vi "Get SSR Status - Multiple.vi"(0 "reference in":refnum<class "SSR.lvclass">, 3 "SSR Channel Numbers (Zero Based)":i32[](array[numeric]), 5 "error in (no error)":errorcluster) -> (14 "reference out":refnum<class "SSR.lvclass">, 17 "SSR Channel Status":bool[](array[boolean]), 19 "error out":errorcluster)   [LabVIEW 2017, in "SSR.lvclass"]
uses:
  SSR.lvclass
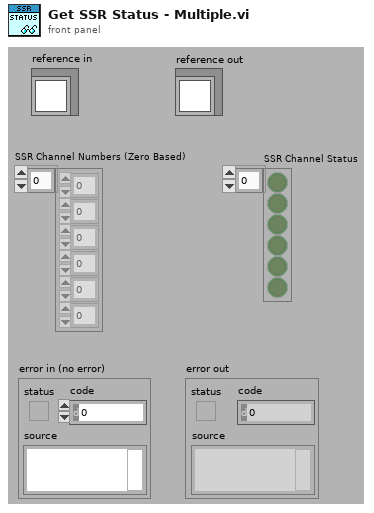
[diagram p1: front panel]
types:
  T1 = typedef "SSR.lvclass/ObjectAttributes.ctl" = cluster{"SSR Task":refnum<k21>, "SSR On/Off Status":bool, "Number of SSR Modules":u32, "Number of Total SSR Channels":u32, "SSR Module Names (NI-Max Name)":string[], "Number of Channels Per SSR Module":i32[], "SSR Status":bool[], "SSR Status to Set":bool[], "SSR VI Reference":refnum<vi>}
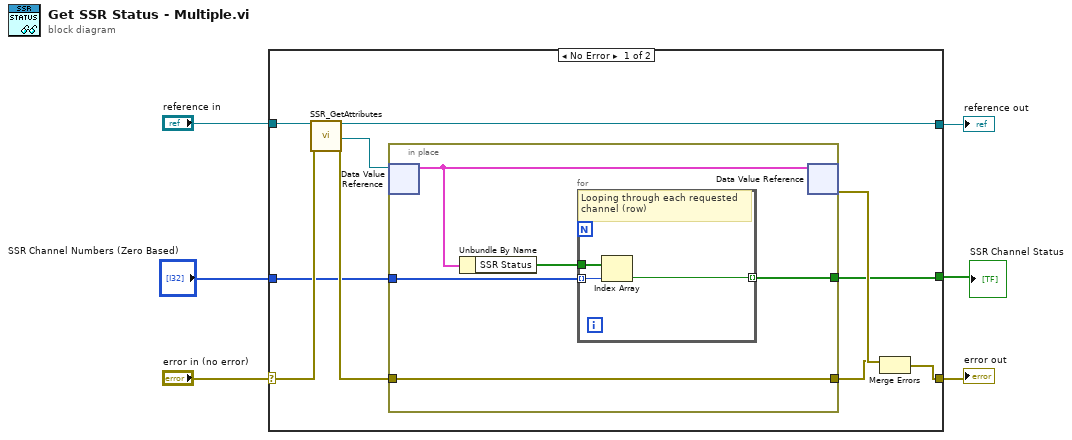
[diagram p0: block diagram]
diagram:
  n1 = case shown="No Error" "error in (no error)" {
    selector: "error in (no error)" -> [w15 w26]
    tunnel: [w12 w26] -> w5
    tunnel: [w13 w25] -> w3
    tunnel: "reference in" -> [w16 w25]
    tunnel: "SSR Channel Numbers (Zero Based)" -> [w8 _]
    tunnel: [w7 _] -> w1
    frame No Error {
      n2 = call "SSR_GetAttributes.vi"("reference in"=w16, "error in (no error)"=w15) -> ("reference out"=w13:refnum<class "SSR.lvclass">, "DataRef"=w11:refnum<data-value>, "error out"=w10:errorcluster)  [unwired: 14 in, 1 out]
      n3 = in-place {
        in-place-border: w10 -> [w21]
        in-place-border: [w21] -> w9
        in-place-border: w8 -> [w18]
        in-place-border: [w17] -> w7
        n4 = in-place-dvr #1(w11) -> (w20:T1)  [unwired: 1 out]
        n5 = Unbundle By Name(w20) -> ("SSR Status"=w19:bool[])
        n6 = for {
          tunnel: w19 -> [w24]
          tunnel: w18 -> [w23] mode=indexing
          tunnel: [w22] -> w17 mode=indexing
          # "Looping through each requested channel (row)"
          n7 = Index Array(array=w24, index=w23) -> (element=w22:bool)
        }
        n8 = in-place-dvr #1(w20) -> (w14:errorcluster)  [unwired: 1 out]
      }
      n9 = Merge Errors(w14, w9) -> (w12:errorcluster)
    }
    frame Error {
    }
  }
  "error out" <- w5
  "reference out" <- w3
  "SSR Channel Status" <- w1
